vi "safeties.vi"(10 "Prev Iteration Data":T5) -> (0 "Safety Data and Log":T5, 1 "Shooter":T1, 2 "Ramp Belts":T2, 3 "Arm Actuator":T3, 5 "Drive Train":T4)   [LabVIEW 2015]
uses:
  <vilib>/Rock Robotics/Network Tables/NT Read Boolean.vi
panel:
  out "Safety Data":bool[][](array[boolean])
  out "Multicolumn Listbox":i32(listbox)
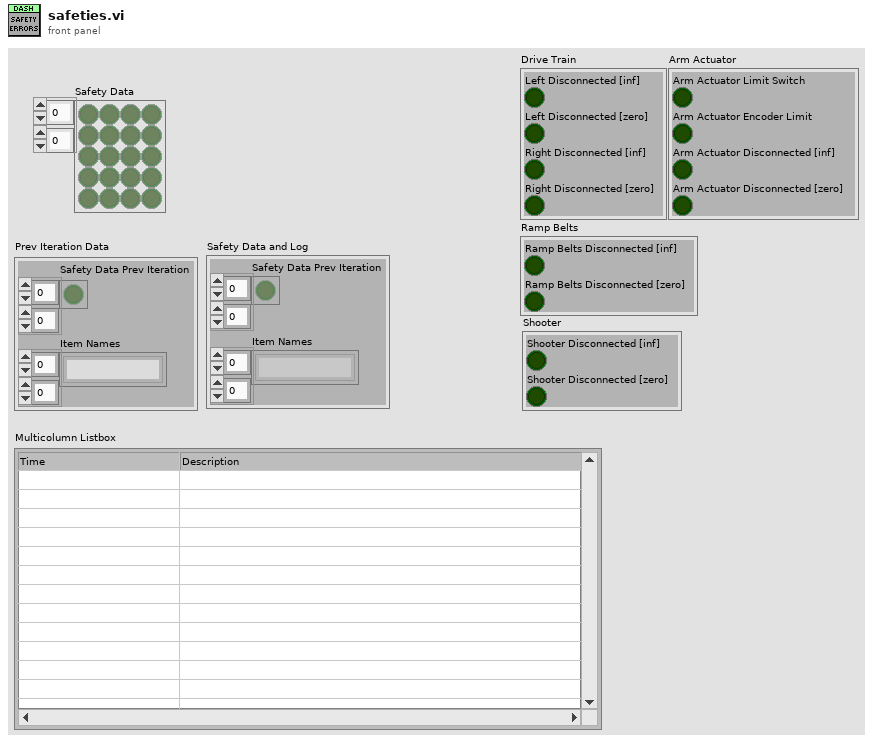
[diagram p1: front panel]
types:
  T1 = cluster{"Shooter Disconnected [inf]":bool, "Shooter Disconnected [zero]":bool}
  T2 = cluster{"Ramp Belts Disconnected [inf]":bool, "Ramp Belts Disconnected [zero]":bool}
  T3 = cluster{"Arm Actuator Limit Switch":bool, "Arm Actuator Encoder Limit":bool, "Arm Actuator Disconnected [inf]":bool, "Arm Actuator Disconnected [zero]":bool}
  T4 = cluster{"Left Disconnected [inf]":bool, "Left Disconnected [zero]":bool, "Right Disconnected [inf]":bool, "Right Disconnected [zero]":bool}
  T5 = cluster{"Safety Data Prev Iteration":bool[][], "Item Names":string[][]}
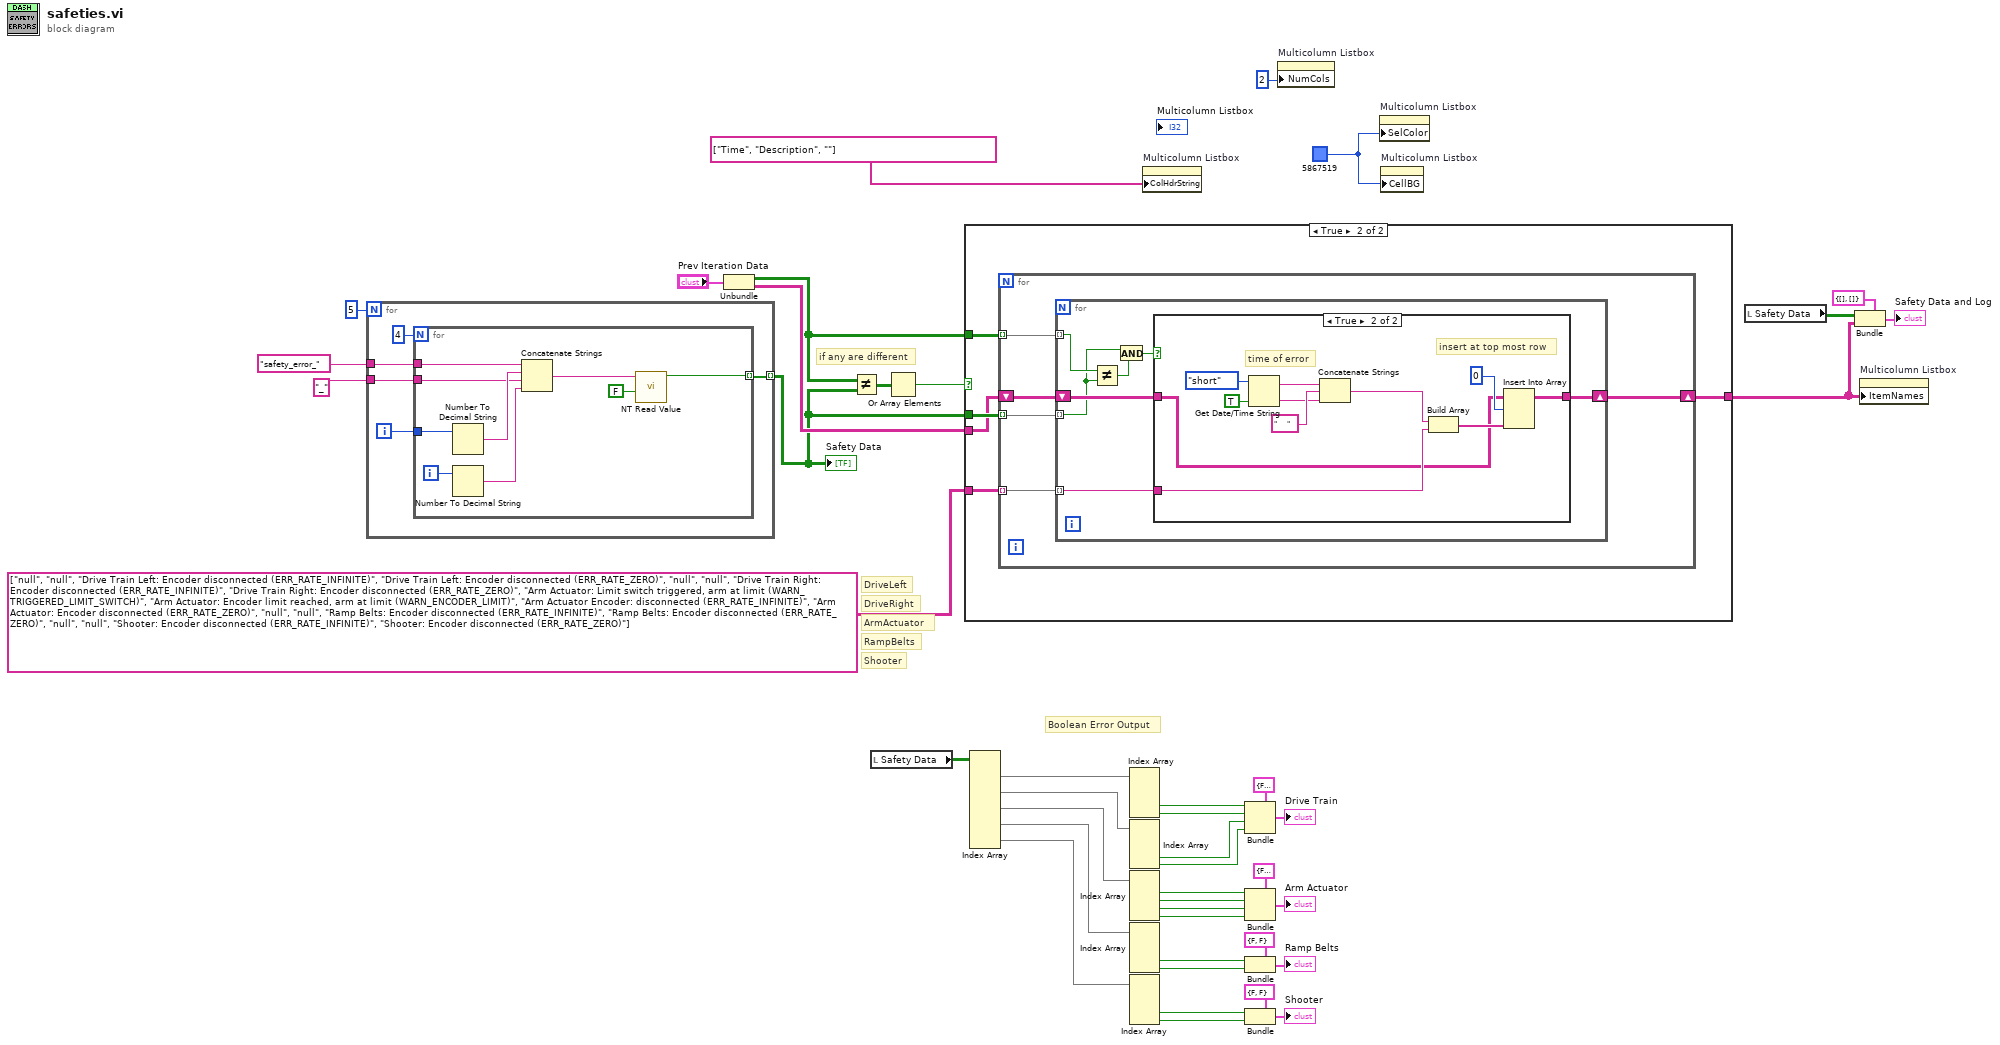
[diagram p0: block diagram]
diagram:
  w34 = u32 5867519 ("Round Color Box")
  # "Boolean Error Output"
  # "Shooter"
  # "RampBelts"
  # "ArmActuator"
  # "DriveRight"
  # "DriveLeft"
  # "if any are different"
  n1 = for {
    N: 5 -> [_]
    tunnel: "safety_error_" ("Name") -> [w47]
    tunnel: "_" ("Name") -> [w46]
    tunnel: [w44] -> w30 mode=indexing
    i -> [w45]
    n2 = for {
      N: 4 -> [_]
      tunnel: w47 -> [w55]
      tunnel: w46 -> [w53]
      tunnel: w45 -> [w57]
      tunnel: [w50] -> w44 mode=indexing
      i -> [w56]
      n3 = Number To Decimal String(number=w57) -> (decimal integer string=w54:string)  [unwired: 1 in]
      n4 = Number To Decimal String(number=w56) -> (decimal integer string=w52:string)  [unwired: 1 in]
      n5 = Concatenate Strings(w55, w54, w53, w52) -> (w51:string)
      n6 = call-poly <vilib>:"NT Read Value.vi"("Default Value"=FALSE, "Name"=w51) -> ("Boolean"=w50:bool)  [unwired: 8 in, 1 out]
    }
  }
  "Safety Data" <- w30
  n7 = Unbundle("Prev Iteration Data") -> ("Safety Data Prev Iteration"=w38:bool[][], "Item Names"=w37:string[][])
  n8 = Not Equal?(x=w38, y=w30) -> (x != y?=w40:bool[][])
  n9 = local read "Safety Data"() -> (w26:bool[][])
  n10 = Or Array Elements(Boolean array=w40) -> (logical OR=w39:bool)
  n11 = case shown="True" w39 {
    tunnel: w30 -> [_ w63]
    tunnel: w38 -> [_ w62]
    tunnel: w37 -> [w58 w59]
    tunnel: [w58 w60] -> w35
    tunnel: string[][] [["null", "null", "Drive Train Left: Encoder disconnected (ERR_RATE_INFINITE)", "Drive Train Left: Encoder disconnected (ERR_RATE_ZERO)"], ["null", "null", "Drive Train Right: Encoder disconnected (ERR_RATE_INFINITE)", "Drive Train Right: Encoder disconnected (ERR_RATE_ZERO)"], ["Arm Actuator: Limit switch triggered, arm at limit (WARN_TRIGGERED_LIMIT_SWITCH)", "Arm Actuator: Encoder limit reached, arm at limit (WARN_ENCODER_LIMIT)", "Arm Actuator Encoder: disconnected (ERR_RATE_INFINITE)", "Arm Actuator: Encoder disconnected (ERR_RATE_ZERO)"], ["null", "null", "Ramp Belts: Encoder disconnected (ERR_RATE_INFINITE)", "Ramp Belts: Encoder disconnected (ERR_RATE_ZERO)"], ["null", "null", "Shooter: Encoder disconnected (ERR_RATE_INFINITE)", "Shooter: Encoder disconnected (ERR_RATE_ZERO)"]] -> [_ w61]
    frame False {
    }
    frame True {
      n12 = for {
        tunnel: w63 -> [w67] mode=indexing
        tunnel: w62 -> [w68] mode=indexing
        tunnel: w61 -> [w66] mode=indexing
        shift-right: [w65] -> w60
        shift-left: w59 -> [w64]
        n13 = for {
          tunnel: w68 -> [w75] mode=indexing
          tunnel: w67 -> [w69] mode=indexing
          tunnel: w66 -> [w74] mode=indexing
          shift-right: [w73] -> w65
          shift-left: w64 -> [w72]
          n14 = Not Equal?(x=w75, y=w69) -> (x != y?=w71:bool)
          n15 = And(x=w69, y=w71) -> (x .and. y?=w70:bool)
          n16 = case shown="True" w70 {
            tunnel: w74 -> [_ w79]
            tunnel: [w76 w78] -> w73
            tunnel: w72 -> [w76 w77]
            frame False {
            }
            frame True {
              # "insert at top most row"
              # "time of error"
              n17 = Get Date/Time String(date format (0)=enum16{"short", "long", "abbreviated"}."short", want seconds? (F)=TRUE) -> (date string=w84:string, time string=w83:string)  [unwired: 1 in]
              n18 = Concatenate Strings(w84, "     " ("string"), w83) -> (w80:string)
              n19 = Build Array(w80, w79) -> (w81:string[])
              n20 = Insert Into Array(array=w77, index (row)=0, new element=w81) -> (w78:string[][])  [unwired: 1 in]
            }
          }
        }
      }
    }
  }
  n21 = Index Array(array=w26) -> (element #1=w25:bool[], element #2=w20:bool[], element #3=w19:bool[], element #4=w18:bool[], element #5=w7:bool[])  [unwired: 10 in]
  n22 = Index Array(array=w25) -> (element #3=w17:bool, element #4=w16:bool)  [unwired: 4 in, 2 out]
  n23 = Index Array(array=w20) -> (element #3=w14:bool, element #4=w15:bool)  [unwired: 4 in, 2 out]
  n24 = Index Array(array=w19) -> (element #1=w10:bool, element #2=w11:bool, element #3=w12:bool, element #4=w13:bool)  [unwired: 4 in]
  n25 = Index Array(array=w18) -> (element #3=w9:bool, element #4=w8:bool)  [unwired: 4 in, 2 out]
  n26 = Index Array(array=w7) -> (element #3=w5:bool, element #4=w6:bool)  [unwired: 4 in, 2 out]
  n27 = property on="Multicolumn Listbox" class="MCListbox (strict)"("ColHdrString"=string[] ["Time", "Description", ""] ("Column Header Strings[]")) -> ()  [unwired: 2 in, 2 out]
  n28 = Bundle(cluster=T4 {"Left Disconnected [inf]"=FALSE, "Left Disconnected [zero]"=FALSE, "Right Disconnected [inf]"=FALSE, "Right Disconnected [zero]"=FALSE}, "Left Disconnected [inf]"=w17, "Left Disconnected [zero]"=w16, "Right Disconnected [inf]"=w14, "Right Disconnected [zero]"=w15) -> (→"Drive Train":T4)
  n29 = Bundle(cluster=T3 {"Arm Actuator Limit Switch"=FALSE, "Arm Actuator Encoder Limit"=FALSE, "Arm Actuator Disconnected [inf]"=FALSE, "Arm Actuator Disconnected [zero]"=FALSE}, "Arm Actuator Limit Switch"=w10, "Arm Actuator Encoder Limit"=w11, "Arm Actuator Disconnected [inf]"=w12, "Arm Actuator Disconnected [zero]"=w13) -> (→"Arm Actuator":T3)
  n30 = Bundle(cluster=T2 {"Ramp Belts Disconnected [inf]"=FALSE, "Ramp Belts Disconnected [zero]"=FALSE}, "Ramp Belts Disconnected [inf]"=w9, "Ramp Belts Disconnected [zero]"=w8) -> (→"Ramp Belts":T2)
  n31 = Bundle(cluster=T1 {"Shooter Disconnected [inf]"=FALSE, "Shooter Disconnected [zero]"=FALSE}, "Shooter Disconnected [inf]"=w5, "Shooter Disconnected [zero]"=w6) -> (→"Shooter":T1)
  n32 = property on="Multicolumn Listbox" class="MCListbox (strict)"("NumCols"=u32 2 ("Number of Columns")) -> ()  [unwired: 2 in, 2 out]
  n33 = property on="Multicolumn Listbox" class="MCListbox (strict)"("SelColor"=w34) -> ()  [unwired: 2 in, 2 out]
  n34 = property on="Multicolumn Listbox" class="MCListbox (strict)"("CellBG"=w34) -> ()  [unwired: 2 in, 2 out]
  n35 = local read "Safety Data"() -> (w28:bool[][])
  n36 = Bundle(cluster=T5 {"Safety Data Prev Iteration"=[], "Item Names"=[]} ("Prev Iteration Data"), "Safety Data Prev Iteration"=w28, "Item Names"=w35) -> (→"Safety Data and Log":T5)
  n37 = property on="Multicolumn Listbox" class="MCListbox (strict)"("ItemNames"=w35) -> ()  [unwired: 2 in, 2 out]
